vi "(SubVI) AutoGain.vi"(8 "error in (no error)":errorcluster, 10 "AutoMode":enum16{"None", "Auto Once", "Continuous"}(ring), 11 "Refnum in":T1) -> (0 "error out":errorcluster, 3 "Refnum out":T1)   [LabVIEW 2014]
uses:
  <vilib>/userdefined/High Color/IMAQdx.ctl
  <resource>/objmgr/imaqdx.rc
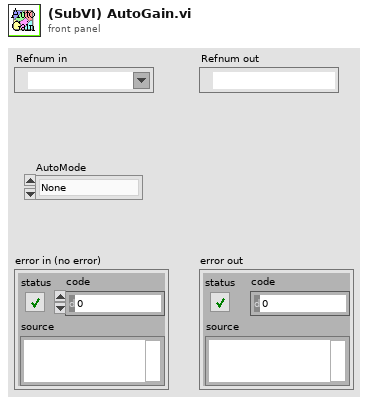
[diagram p1: front panel]
types:
  T1 = typedef "IMAQdx.ctl" = refnum<k21>
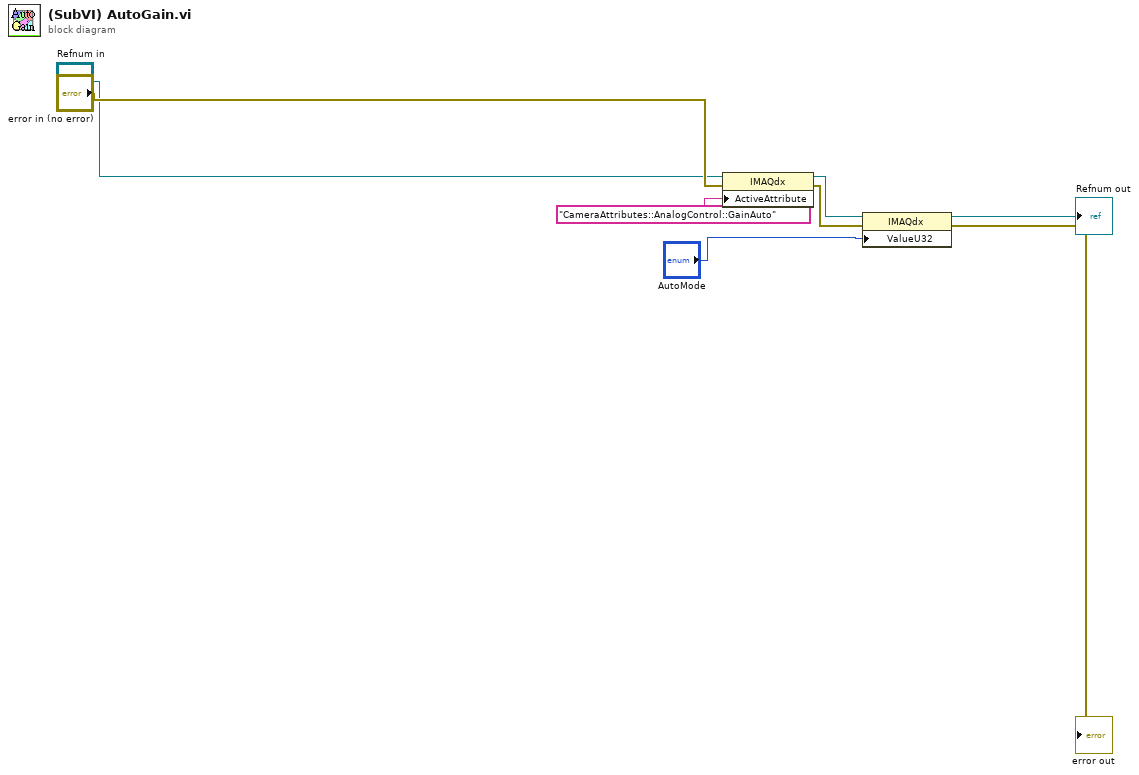
[diagram p0: block diagram]
diagram:
  n1 = property class="IMAQdx"(reference="Refnum in", error in="error in (no error)", "ActiveAttribute"="CameraAttributes::AnalogControl::GainAuto") -> (reference out=w2:T1, error out=w3:errorcluster)
  n2 = property class="IMAQdx"(reference=w2, error in=w3, "ValueU32"="AutoMode") -> (reference out=→"Refnum out":T1, error out=→"error out":errorcluster)
